vi "Run Secondary VI(SubVI).vi"(8 "error in (no error)":errorcluster, 11 "Secondary VI":u16) -> (0 "error out":errorcluster)   [LabVIEW 2014]
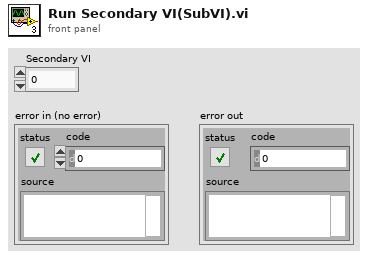
[diagram p1: front panel]
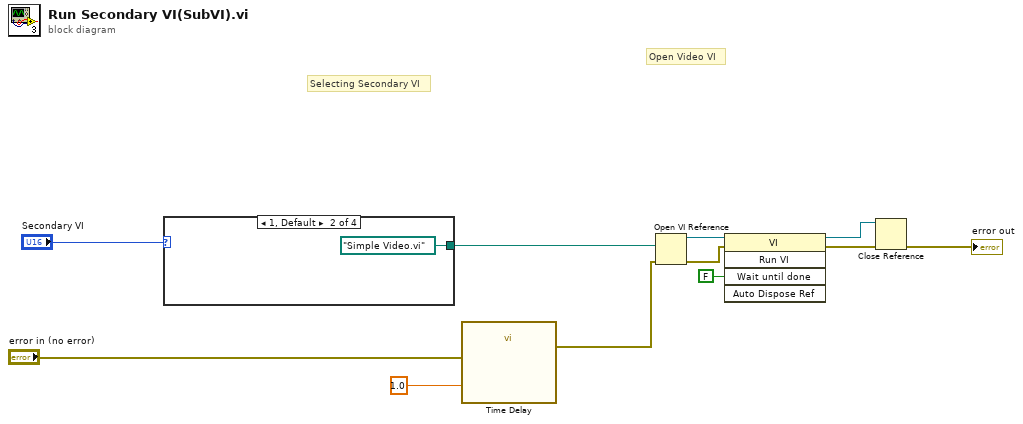
[diagram p0: block diagram]
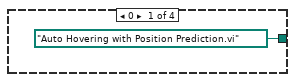
[diagram p2: hidden frame]
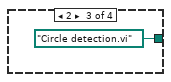
[diagram p3: hidden frame]
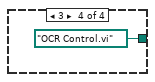
[diagram p4: hidden frame]
diagram:
  # "Selecting Secondary VI"
  # "Open Video VI"
  n1 = case shown="1, Default" "Secondary VI" {
    tunnel: [path "Auto Hovering with Position Prediction.vi" ("Video Acquisition VI path") path "Simple Video.vi" ("Video Acquisition VI path") path "Circle detection.vi" ("Video Acquisition VI path") path "OCR Control.vi" ("Video Acquisition VI path")] -> w6
    frame 0 {
    }
    frame 1, Default {
    }
    frame 2 {
    }
    frame 3 {
    }
  }
  n2 = call "Time Delay"("error in (no error)"="error in (no error)", "Delay Time (s)"=1.0) -> ("error out"=w9:errorcluster)  [unwired: 9 in]
  n3 = Open VI Reference(vi path=w6, error in (no error)=w9) -> (vi reference=w4:refnum<vi>, error out=w1:errorcluster)  [unwired: 4 in]
  n4 = invoke class="VI" method="Run VI"(reference=w4, error in=w1, "Wait until done"=FALSE) -> (reference out=w3:refnum<vi>, error out=w11:errorcluster)  [unwired: 2 in, 3 out]
  n5 = Close Reference(reference=w3, error in (no error)=w11) -> (error out=→"error out":errorcluster)
